vi "testa get last camera data.vi"() -> ()   [LabVIEW 2016]
uses:
  GitHub/SSLView/SSL Detection Frame.ctl
  GitHub/SSLView/SSL Detection Robot.ctl
  GitHub/SSLView/SSL Detection Ball.ctl
  <vilib>/Utility/tcp.llb/UDP Multicast Read-Only Open.vi
panel:
  in  "life time":dbl=1.0 format="%#_13g"
  out "LAST DATA":T1(array[cluster])
  in  "camera_id":u32
  in  "Now":timestamp
  in  "stop":bool
  out "Detection Frame Out":T2
  out "error out":errorcluster
  in  "port":u16
  in  "String":string
  # "testa get last camera data\nabre comunicação UDP pela porta\nem que o ssl-vision está jogando os dados das câmeras"
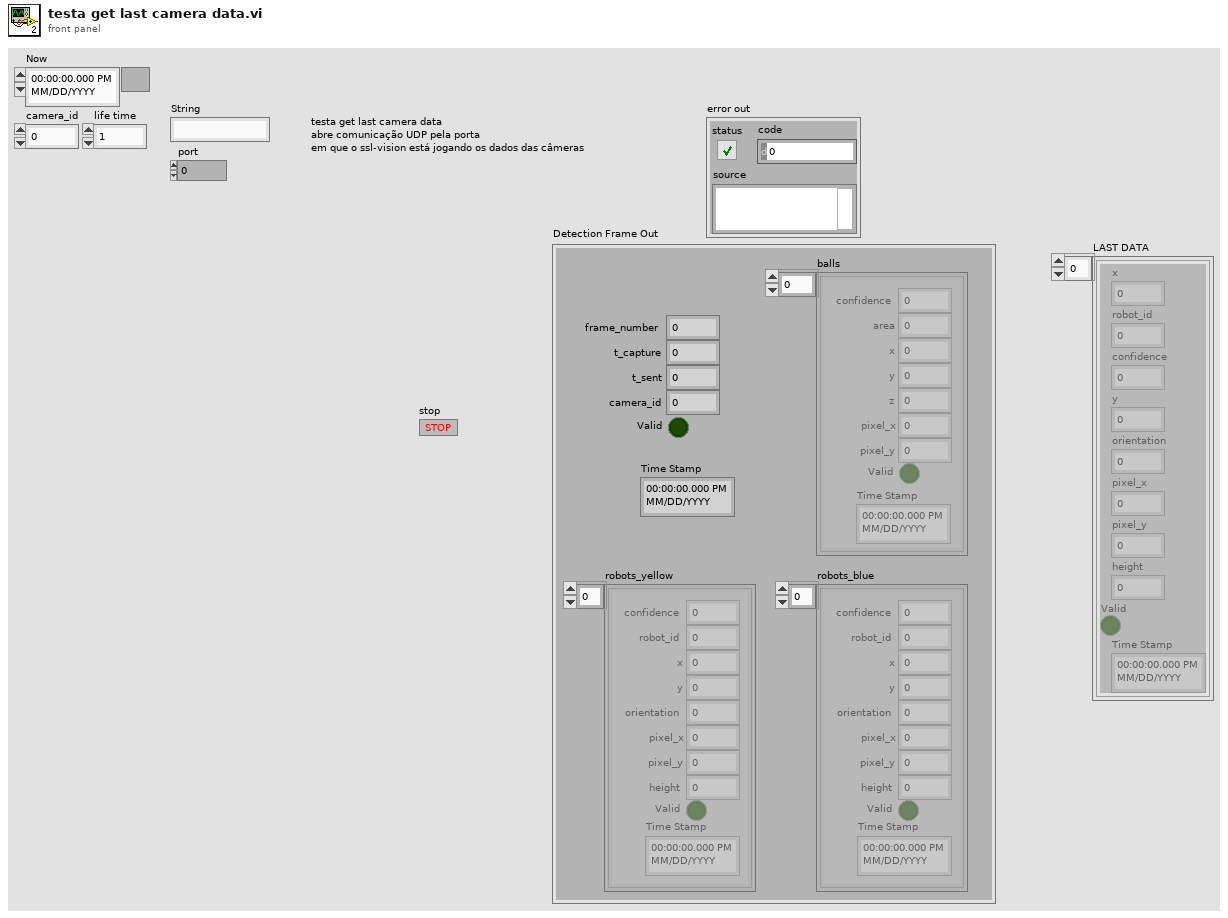
[diagram p1: front panel]
types:
  T1 = cluster{"x":dbl, "robot_id":u32, "confidence":sgl, "y":sgl, "orientation":sgl, "pixel_x":sgl, "pixel_y":sgl, "height":sgl, "Valid":bool, "Time Stamp":timestamp}[]
  T2 = typedef "SSL Detection Frame.ctl" = cluster{"frame_number":u32, "t_capture":dbl, "t_sent":dbl, "camera_id":u32, "robots_yellow":T3[], "robots_blue":T3[], "balls":T4[], "Valid":bool, "Time Stamp":timestamp}
  T3 = typedef "SSL Detection Robot.ctl" = cluster{"x":dbl, "robot_id":u32, "confidence":sgl, "y":sgl, "orientation":sgl, "pixel_x":sgl, "pixel_y":sgl, "height":sgl, "Valid":bool, "Time Stamp":timestamp}
  T4 = typedef "SSL Detection Ball.ctl" = cluster{"x":sgl, "area":u32, "confidence":sgl, "y":sgl, "z":sgl, "pixel_x":sgl, "pixel_y":sgl, "Valid":bool, "Time Stamp":timestamp}
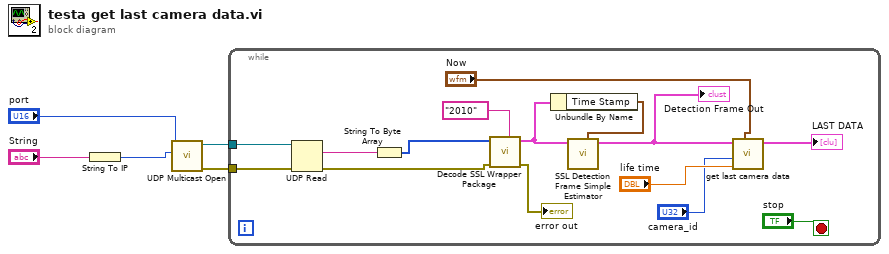
[diagram p0: block diagram]
diagram:
  n1 = String To IP(1:"String") -> (0:w4:u32)
  n2 = call-poly <vilib>:"UDP Multicast Open.vi"("multicast addr"=w4, "port"="port") -> ("error out"=w1:errorcluster, "connection ID"=w2:refnum<k16>)  [unwired: 7 in, 1 out]
  n3 = while {
    tunnel: w2 -> [w20]
    tunnel: w1 -> [w19]
    stop <- "stop" stop-if-true
    n4 = UDP Read(connection ID=w20, 8:w19) -> (data out=w18:string, error out=w16:errorcluster)  [unwired: 2 in, 3 out]
    n5 = String To Byte Array(string=w18) -> (unsigned byte array=w17:u8[])
    n6 = call "Decode SSL Wrapper Package.vi"("Version"="2010", "error in (no error)"=w16, "unsigned byte array"=w17) -> ("error out"=→"error out":errorcluster, "Detection Frame"=w13:T2)  [unwired: 5 in, 2 out]
    n7 = Unbundle By Name(w13) -> ("Time Stamp"=w12:timestamp)
    n8 = call "SSL Detection Frame Simple Estimator.vi"("Now"=w12, "Detection Frame In"=w13) -> ("Detection Frame Out"=w7:T2)  [unwired: 9 in]
    "Detection Frame Out" <- w7
    n9 = call "get last camera data.vi"("Now"="Now", "life time"="life time", "camera_id"="camera_id", "Detection Frame In"=w7) -> ("output array"=→"LAST DATA":T1)  [unwired: 7 in]
  }
